vi "Configure Over Voltage Protection.vi"(8 "error in (no error)":errorcluster, 10 "Voltage Limit (0)":u16(ring) items=["None", "2", "5", "10", "20", "40", "60", "80", "100", "120", "140", "160", "180", "200", "300", "400", "500"], 11 "VISA resource name":refnum<visa-resource-name>) -> (0 "error out":errorcluster, 3 "VISA resource name out":refnum<visa-resource-name>)   [LabVIEW 2018, in "Keithley 2450.lvlib"]
doc: "Sets a maximum voltage on the instrument to prevent overloading devices under test."
uses:
  <instrlib>/Keithley 2450/Keithley 2450.lvlib
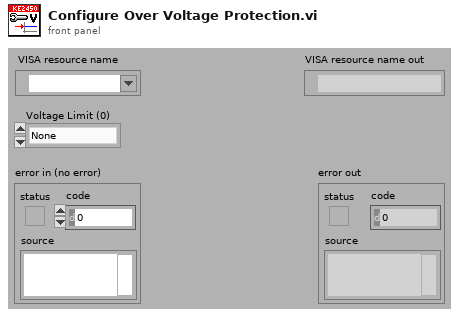
[diagram p1: front panel]
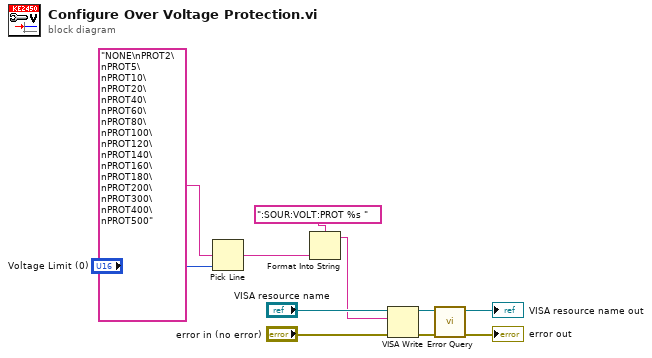
[diagram p0: block diagram]
diagram:
  n1 = Pick Line(multi-line string="NONE\nPROT2\nPROT5\nPROT10\nPROT20\nPROT40\nPROT60\nPROT80\nPROT100\nPROT120\nPROT140\nPROT160\nPROT180\nPROT200\nPROT300\nPROT400\nPROT500", line index="Voltage Limit (0)") -> (output string=w1:string)  [unwired: 1 in]
  n2 = Format Into String(format string=":SOUR:VOLT:PROT %s ", w1) -> (resulting string=w4:string)  [unwired: 2 in, 1 out]
  n3 = VISA Write(VISA resource name="VISA resource name", write buffer=w4, error in (no error)="error in (no error)") -> (VISA resource name out=w7:refnum<visa-resource-name>, error out=w6:errorcluster)  [unwired: 1 out]
  n4 = call <instrlib>:"Error Query.vi"("error in (no error)"=w6, "VISA resource name"=w7) -> ("error out"=→"error out":errorcluster, "VISA resource name out"=→"VISA resource name out":refnum<visa-resource-name>)  [unwired: 8 out]
